vi "Error_Log to File.vi"(7 "Error Log Filepath":path=path "d:/", 8 "error in (no error)":errorcluster, 10 "Error Data_IN":errorcluster, 11 "Error Log Filename":string) -> (0 "error out":errorcluster, 2 "Error Data_OUT":errorcluster, 3 "Error Data (2D String Array)":string[][](array[string]), 5 "Call chain empty?":bool)   [LabVIEW 2019]
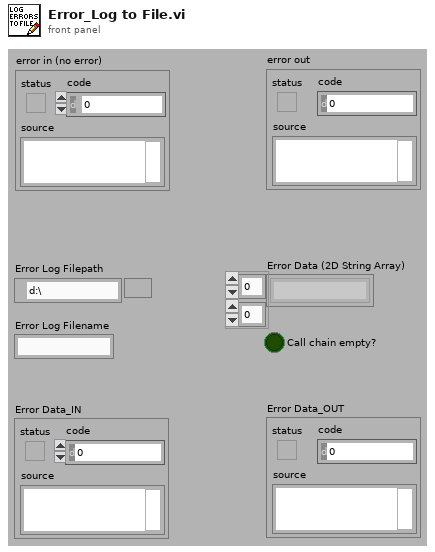
[diagram p1: front panel]
types:
  T1 = enum16{"open", "replace", "create", "open or create", "replace or create", "replace or create with confirmation"}
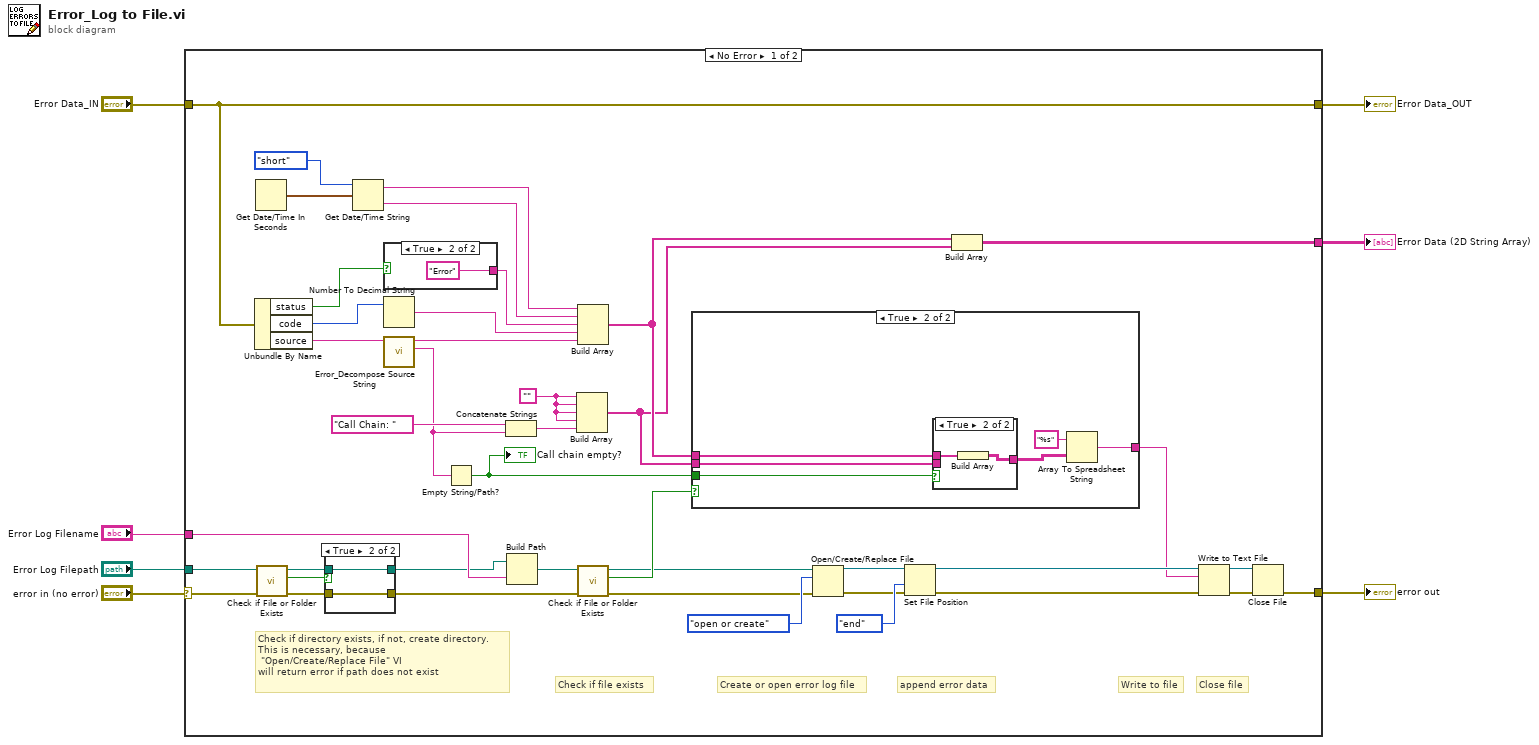
[diagram p0: block diagram]
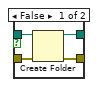
[diagram p2: hidden frame]
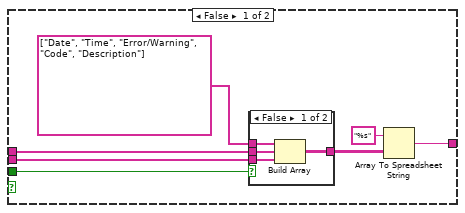
[diagram p3: hidden frame]
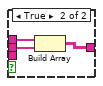
[diagram p4: hidden frame]
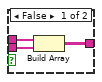
[diagram p5: hidden frame]
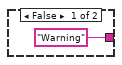
[diagram p6: hidden frame]
diagram:
  n1 = case shown="No Error" "error in (no error)" {
    selector: "error in (no error)" -> [w29 w83]
    tunnel: "Error Log Filepath" -> [w28 _]
    tunnel: [w40 w83] -> w6
    tunnel: "Error Log Filename" -> [w39 _]
    tunnel: "Error Data_IN" -> [w18 w82]
    tunnel: [w12 _] -> w2
    tunnel: [w18 w82] -> w1
    frame No Error {
      w10 = ""
      # "Close file"
      # "Write to file"
      # "Check if file exists"
      # "append error data"
      # "Check if directory exists, if not, create directory.\nThis is necessary, because\n \"Open/Create/Replace File\" VI\nwill return error if path does not exist"
      # "Create or open error log file"
      n2 = Unbundle By Name(w18) -> ("status"=w36:bool, "code"=w38:i32, "source"=w17:string)
      n3 = Get Date/Time In Seconds() -> (seconds since 1Jan1904=w22:timestamp)
      n4 = call <vilib>:"Check if File or Folder Exists.vi"("error in (no error)"=w29, "path"=w28) -> ("error out"=w27:errorcluster, "file or folder exists?"=w24:bool, "dup path"=w25:path)  [unwired: 7 in]
      n5 = case shown="True" w24 {
        tunnel: w27 -> [w52 w54]
        tunnel: [w51 w54] -> w26
        tunnel: w25 -> [w50 w53]
        tunnel: [w49 w53] -> w23
        frame False {
          n6 = Create Folder(path (use dialog)=w50, error in=w52) -> (created path=w49:path, error out=w51:errorcluster)  [unwired: 1 in, 1 out]
        }
        frame True {
        }
      }
      n7 = Get Date/Time String(date format (0)=enum16{"short", "long", "abbreviated"}."short", seconds (now)=w22) -> (date string=w21:string, time string=w20:string)  [unwired: 1 in]
      n8 = case shown="True" w36 {
        tunnel: ["Warning" "Error"] -> w35
        frame False {
        }
        frame True {
        }
      }
      n9 = Number To Decimal String(number=w38) -> (decimal integer string=w37:string)  [unwired: 1 in]
      n10 = call "Error_Decompose Source String.vi"("Error Source (String)"=w17) -> ("Call Chain"=w11:string, "Description"=w16:string)  [unwired: 9 in]
      n11 = Empty String/Path?(string/path=w11) -> (empty?=w8:bool)
      "Call chain empty?" <- w8
      n12 = Concatenate Strings("Call Chain: " ("string"), w11) -> (w9:string)
      n13 = Build Path(base path=w23, name or relative path=w39) -> (appended path=w34:path)
      n14 = Build Array(w10, w10, w10, w10, w9) -> (w13:string[])
      n15 = Build Array(w21, w20, w35, w37, w16) -> (w14:string[])
      n16 = call <vilib>:"Check if File or Folder Exists.vi"("error in (no error)"=w26, "path"=w34) -> ("error out"=w33:errorcluster, "file or folder exists?"=w32:bool, "dup path"=w30:path)  [unwired: 7 in]
      n17 = case shown="True" w32 {
        tunnel: w14 -> [w58 w71]
        tunnel: [w60 w73] -> w31
        tunnel: w13 -> [w56 w70]
        tunnel: w8 -> [w55 w69]
        frame False {
          n18 = case shown="False" w55 {
            tunnel: [w65 w68] -> w59
            tunnel: w58 -> [w64 w67]
            tunnel: string[] ["Date", "Time", "Error/Warning", "Code", "Description"] ("element") -> [w63 w66]
            tunnel: w56 -> [w62 _]
            frame False {
              n19 = Build Array(w63, w64, w62) -> (w65:string[][])
            }
            frame True {
              n20 = Build Array(w66, w67) -> (w68:string[][])
            }
          }
          n21 = Array To Spreadsheet String(array=w59, 3:"%s" ("format string")) -> (spreadsheet string=w60:string)  [unwired: 1 in]
        }
        frame True {
          n22 = case shown="True" w69 {
            tunnel: [w77 w79] -> w72
            tunnel: w71 -> [w76 w78]
            tunnel: w70 -> [w75 _]
            frame False {
              n23 = Build Array(w76, w75) -> (w77:string[][])
            }
            frame True {
              n24 = Build Array(w78) -> (w79:string[][])
            }
          }
          n25 = Array To Spreadsheet String(array=w72, 3:"%s" ("format string")) -> (spreadsheet string=w73:string)  [unwired: 1 in]
        }
      }
      n26 = Open/Create/Replace File(file path (use dialog)=w30, error in=w33, operation (0:open)=T1."open or create") -> (refnum out=w41:refnum<file>, error out=w42:errorcluster)  [unwired: 3 in, 1 out]
      n27 = Set File Position(refnum=w41, from (0:start)=enum16{"start", "end", "current"}."end", error in=w42) -> (refnum out=w46:refnum<file>, error out=w45:errorcluster)  [unwired: 1 in]
      n28 = Build Array(w14, w13) -> (w12:string[][])
      n29 = Write to Text File(file (use dialog)=w46, text=w31, error in=w45) -> (refnum out=w48:refnum<file>, error out=w47:errorcluster)  [unwired: 1 in, 1 out]
      n30 = Close File(refnum=w48, error in=w47) -> (error out=w40:errorcluster)  [unwired: 1 out]
    }
    frame Error {
    }
  }
  "error out" <- w6
  "Error Data (2D String Array)" <- w2
  "Error Data_OUT" <- w1
